vi "JSON Flatten.vi"(4 "Enums as string? (F)":bool, 6 "Pretty Print? (F)":bool, 8 "error in (no error)":errorcluster, 10 "Root Path ([]=Root)":string[](array[string]), 11 "Variant in":variant) -> (0 "error out":errorcluster, 3 "JSON out":string)   [LabVIEW 2019, in "labview_json.lvlib"]
doc: "Exports a <b>Variant</b> to a <b>JSON</b> string. Set <b>Enums as string?</b> to True to export enums as a string, otherwise enums are considered unsigned integers. Set <b>Pretty Print?</b> to True to add indentation to the output JSON string.\nCreated by: Ryan Pacini"
uses:
  labview_json.lvlib
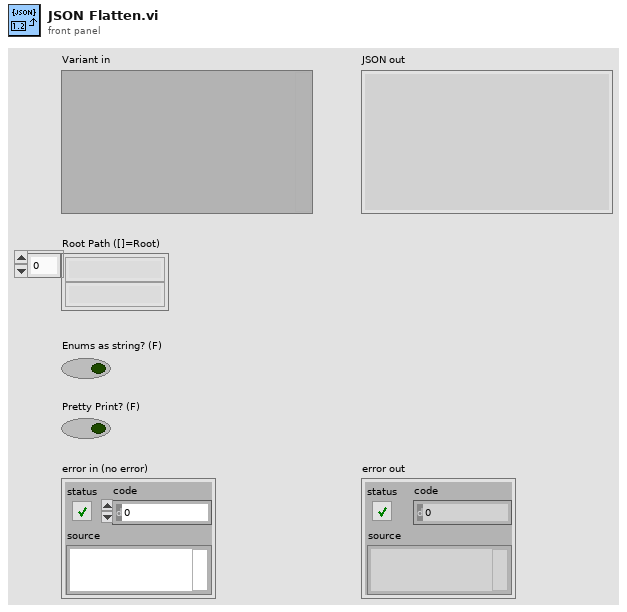
[diagram p1: front panel]
types:
  T1 = typedef "labview_json.lvlib/Element.ctl" = cluster{"Key":string, "Type":T2, "Value":variant}
  T2 = typedef "labview_json.lvlib/Element Type.ctl" = enum8{"NULL", "BOOL", "INT", "UINT", "FLOAT", "STRING", "ARRAY", "OBJECT", "SKIP"}
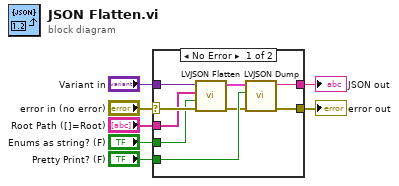
[diagram p0: block diagram]
diagram:
  n1 = case shown="No Error" "error in (no error)" {
    selector: "error in (no error)" -> [w16 w17]
    tunnel: "Variant in" -> [w15 _]
    tunnel: [w13 w17] -> w5
    tunnel: "Enums as string? (F)" -> [w10 _]
    tunnel: [w12 _] -> w3
    tunnel: "Pretty Print? (F)" -> [w11 _]
    tunnel: "Root Path ([]=Root)" -> [w8 _]
    frame No Error {
      n2 = call "LVJSON Flatten.vi"("error in (no error)"=w16, "Enums as string? (F)"=w10, "Root Path ([]=Root)"=w8, "Variant in"=w15) -> ("error out"=w9:errorcluster, "Root Element out"=w14:T1)  [unwired: 6 in]
      n3 = call "LVJSON Dump.vi"("error in (no error)"=w9, "Pretty Print? (F)"=w11, "Root Element in"=w14) -> ("error out"=w13:errorcluster, "JSON out"=w12:string)  [unwired: 6 in, 1 out]
    }
    frame Error {
    }
  }
  "error out" <- w5
  "JSON out" <- w3
